vi "CIMAQ_UniqueString.vi"() -> (1 "String":string)   [LabVIEW 2017]
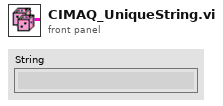
[diagram p1: front panel]
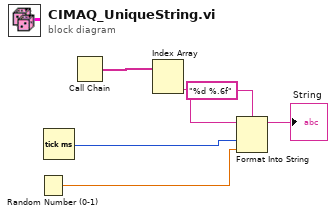
[diagram p0: block diagram]
diagram:
  n1 = Random Number (0-1)() -> (number: 0 to 1=w1:dbl)
  n2 = Tick Count (ms)() -> (millisecond timer value=w3:u32)
  n3 = Call Chain() -> (call chain=w6:string[])
  n4 = Index Array "Index Array"(array=w6) -> (element #2=w2:string)  [unwired: 2 in, 1 out]
  n5 = Format Into String(format string="%d %.6f", initial string=w2, w3, w1) -> (resulting string=→"String":string)  [unwired: 1 in, 1 out]
